vi "FTW-JSON-Interpret.vi"(5 "JSON String":string, 9 "Starting Offset":i32, 11 "error in":errorcluster) -> (4 "Data Name":string, 6 "JSON Type":T1, 8 "Variant Type and Value":variant, 10 "Offset after Match":i32, 15 "error out":errorcluster)   [LabVIEW 2015]
uses:
  FTW-JSON-Type.ctl
panel:
  out "Match":string
  out "Found Match?":bool
  # "Inputs"
  # "Outputs"
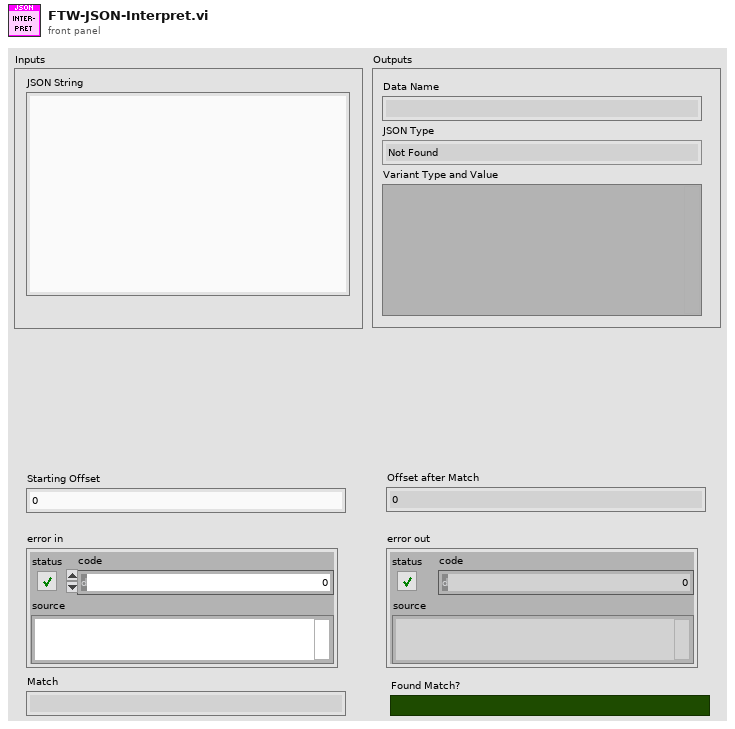
[diagram p1: front panel]
types:
  T1 = typedef "FTW-JSON-Type.ctl" = enum8{"Not Found", "Object", "Array", "String", "Number", "Boolean", "null"}
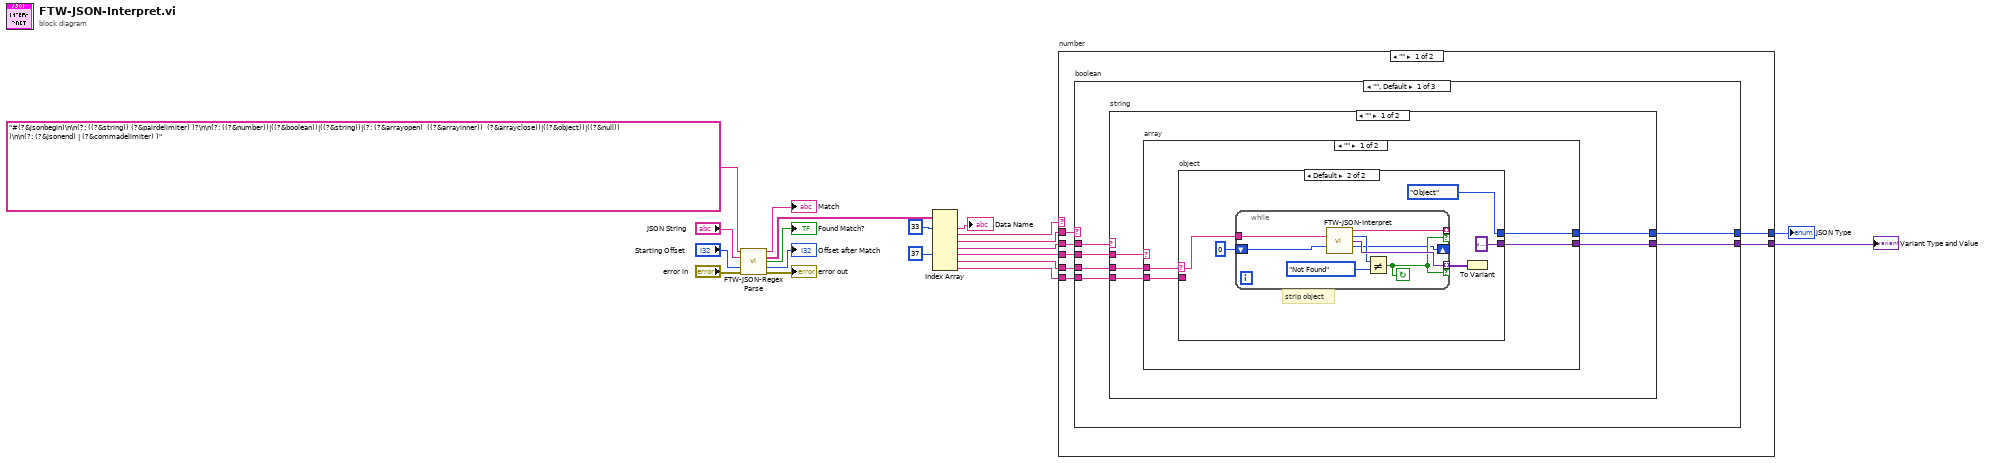
[diagram p0: block diagram]
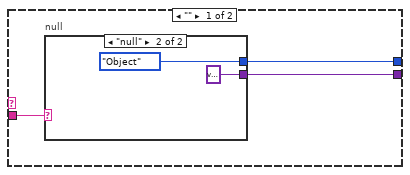
[diagram p2: hidden frame]
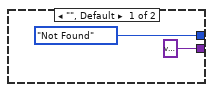
[diagram p3: hidden frame]
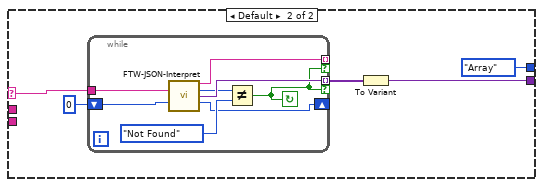
[diagram p4: hidden frame]
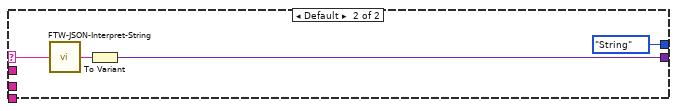
[diagram p5: hidden frame]
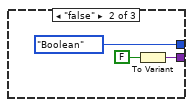
[diagram p6: hidden frame]
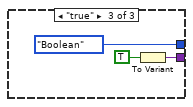
[diagram p7: hidden frame]
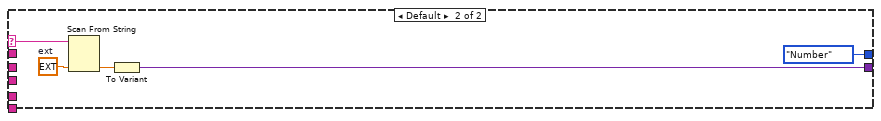
[diagram p8: hidden frame]
diagram:
  n1 = call "FTW-JSON-RegexParse.vi"("Regular Expression using JSON subroutines"="#(?&jsonbegin)\n\n(?: ((?&string)) (?&pairdelimiter) )?\n\n(?: ((?&number))|((?&boolean))|((?&string))|(?: (?&arrayopen)  ((?&arrayinner))  (?&arrayclose))|((?&object))|((?&null)) )\n\n(?: (?&jsonend) | (?&commadelimiter) )", "Input String"="JSON String", "Starting Offset"="Starting Offset", "error in"="error in") -> ("Match"=→"Match":string, "Submatches"=w20:string[], "Found Match?"=→"Found Match?":bool, "Offset after Match"=→"Offset after Match":i32, "error out"=→"error out":errorcluster)  [unwired: 7 in]
  n2 = Index Array(array=w20, index #1=33 ("index"), index #5=37 ("index")) -> (element #1=→"Data Name":string, element #2=w11:string, element #3=w9:string, element #4=w7:string, element #5=w6:string, element #6=w5:string, element #7=w4:string)  [unwired: 5 in]
  n3 = case "number" shown="\"\"" w11 {
    selector: w11 -> [_ w87]
    tunnel: [w27 FTW-JSON-Type."Number" ("JSON Type")] -> w10
    tunnel: w9 -> [w26 _]
    tunnel: [w25 w88] -> w8
    tunnel: w7 -> [w24 _]
    tunnel: w6 -> [w23 _]
    tunnel: w5 -> [w22 _]
    tunnel: w4 -> [w21 _]
    frame "" {
      n4 = case "boolean" shown="\"\", Default" w26 {
        tunnel: [w33 FTW-JSON-Type."Boolean" ("JSON Type") FTW-JSON-Type."Boolean" ("JSON Type")] -> w27
        tunnel: [w31 w80 w83] -> w25
        tunnel: w24 -> [w32 _ _]
        tunnel: w23 -> [w30 _ _]
        tunnel: w22 -> [w29 _ _]
        tunnel: w21 -> [w28 _ _]
        frame "", Default {
          n5 = case "string" shown="\"\"" w32 {
            selector: w32 -> [_ w78]
            tunnel: [w37 FTW-JSON-Type."String" ("JSON Type")] -> w33
            tunnel: [w36 w76] -> w31
            tunnel: w30 -> [w38 _]
            tunnel: w29 -> [w35 _]
            tunnel: w28 -> [w34 _]
            frame "" {
              n6 = case "array" shown="\"\"" w38 {
                selector: w38 -> [_ w66]
                tunnel: [w42 FTW-JSON-Type."Array" ("JSON Type")] -> w37
                tunnel: [w41 w64] -> w36
                tunnel: w35 -> [w40 _]
                tunnel: w34 -> [w39 _]
                frame "" {
                  n7 = case "object" shown="Default" w40 {
                    selector: w40 -> [_ w50]
                    tunnel: [w44 FTW-JSON-Type."Object" ("JSON Type")] -> w42
                    tunnel: [w45 variant] -> w41
                    tunnel: w39 -> [w43 _]
                    frame "" {
                      n8 = case "null" shown="\"null\"" w43 {
                        tunnel: [FTW-JSON-Type."Not Found" ("JSON Type") FTW-JSON-Type."Object" ("JSON Type")] -> w44
                        tunnel: [variant variant] -> w45
                        frame "", Default {
                        }
                        frame "null" {
                        }
                      }
                    }
                    frame Default {
                      # "strip object"
                      n9 = while {
                        tunnel: w50 -> [w62]
                        tunnel: [w61] -> _ mode=indexing if=w57
                        tunnel: [w60] -> w52 mode=indexing if=w57
                        shift-right: [w55] -> _
                        shift-left: 0 -> [w56]
                        stop <- w57 continue-if-true
                        n10 = call "FTW-JSON-Interpret.vi"("JSON String"=w62, "Starting Offset"=w56) -> ("Data Name"=w61:string, "JSON Type"=w59:T1, "Variant Type and Value"=w60:variant, "Offset after Match"=w55:i32)  [unwired: 9 in, 1 out]
                        n11 = Not Equal?(x=w59, y=FTW-JSON-Type."Not Found") -> (x != y?=w57:bool)
                      }
                      n12 = To Variant(anything=w52) -> ()  [unwired: 1 out]
                    }
                  }
                }
                frame Default {
                  n13 = while {
                    tunnel: w66 -> [w75]
                    tunnel: [w74] -> _ mode=indexing if=w70
                    tunnel: [w73] -> w65 mode=indexing if=w70
                    shift-right: [w68] -> _
                    shift-left: 0 -> [w69]
                    stop <- w70 continue-if-true
                    n14 = call "FTW-JSON-Interpret.vi"("JSON String"=w75, "Starting Offset"=w69) -> ("Data Name"=w74:string, "JSON Type"=w72:T1, "Variant Type and Value"=w73:variant, "Offset after Match"=w68:i32)  [unwired: 9 in, 1 out]
                    n15 = Not Equal?(x=w72, y=FTW-JSON-Type."Not Found") -> (x != y?=w70:bool)
                  }
                  n16 = To Variant(anything=w65) -> (Variant=w64:variant)
                }
              }
            }
            frame Default {
              n17 = call "FTW-JSON-Interpret-String.vi"("JSON String"=w78) -> ("LabVIEW String"=w77:string)
              n18 = To Variant(anything=w77) -> (Variant=w76:variant)
            }
          }
        }
        frame "false" {
          n19 = To Variant(anything=FALSE) -> (Variant=w80:variant)
        }
        frame "true" {
          n20 = To Variant(anything=TRUE) -> (Variant=w83:variant)
        }
      }
    }
    frame Default {
      w86 = ext 0.0  # ext
      n21 = Scan From String(input string=w87, default 1=w86) -> (output 1=w89:ext)  [unwired: 3 in, 3 out]
      n22 = To Variant(anything=w89) -> (Variant=w88:variant)
    }
  }
  "JSON Type" <- w10
  "Variant Type and Value" <- w8
